vi "Close Instrument.vi"(0 "RFSG Handle":refnum<k15>, 11 "error in (no error)":errorcluster) -> (15 "error out":errorcluster)   [LabVIEW 2019, in "SG.lvlib"]
doc: "Aborts generation, disables the output, and closes the instrument session."
uses:
  SG.lvlib
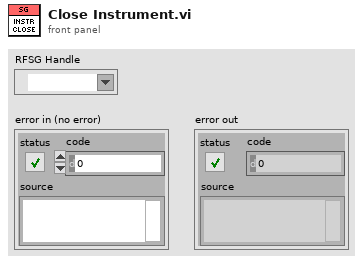
[diagram p1: front panel]
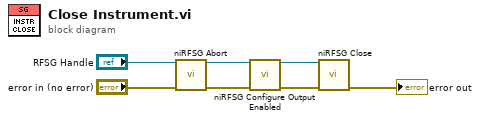
[diagram p0: block diagram]
diagram:
  n1 = call <instrlib>:"niRFSG Abort.vi"("instrument handle"="RFSG Handle", "error in"="error in (no error)") -> ("instrument handle out"=w5:refnum<k15>, "error out"=w7:errorcluster)  [unwired: 12 in]
  n2 = call <instrlib>:"niRFSG Configure Output Enabled.vi"("instrument handle"=w5, "error in"=w7) -> ("instrument handle out"=w4:refnum<k15>, "error out"=w6:errorcluster)  [unwired: 12 in]
  n3 = call <instrlib>:"niRFSG Close.vi"("instrument handle"=w4, "error in"=w6) -> ("error out"=→"error out":errorcluster)  [unwired: 13 in]
